vi "Open.vi"(7 "Config data in":variant, 8 "error in (no error)":errorcluster, 9 "Timeout (ms)":u32=3000, 10 "VISA session":refnum<visa-resource-name>="TCPIP::146.201.232.88::7180::SOCKET", 11 "PS Driver.lvlib:PS Driver.lvclass in":refnum<class "PS Driver.lvclass">) -> (0 "error out":errorcluster, 1 "Config data out":variant, 2 "dup VISA Session":refnum<visa-resource-name>, 3 "PS Driver.lvlib:PS Driver.lvclass out":refnum<class "PS Driver.lvclass">)   [LabVIEW 2020, in "PS Driver.lvlib" / "PS Driver.lvclass"]
uses:
  PS Driver.lvclass
  PS Driver.lvclass/PS Driver.ctl
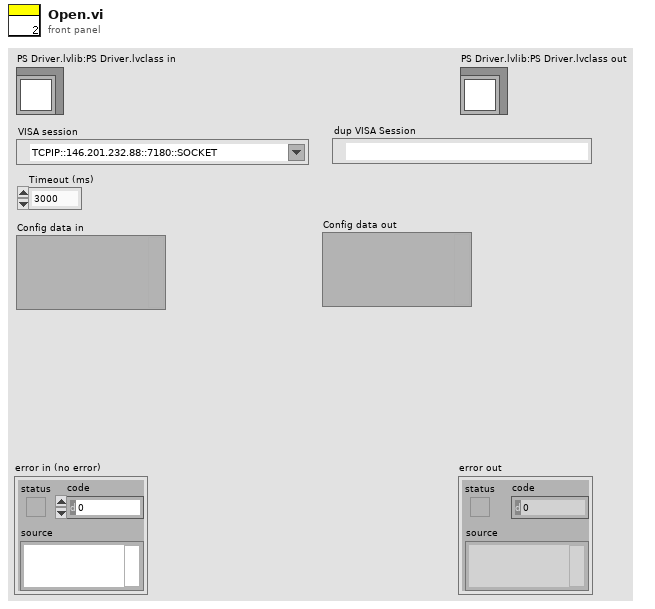
[diagram p1: front panel]
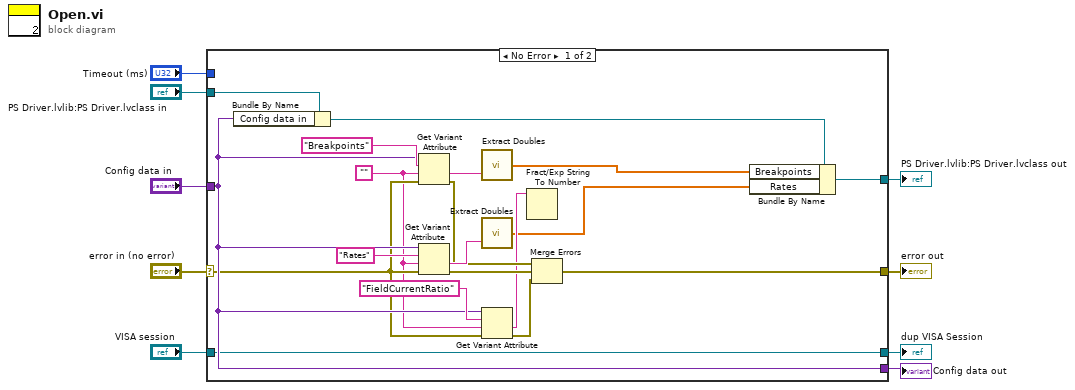
[diagram p0: block diagram]
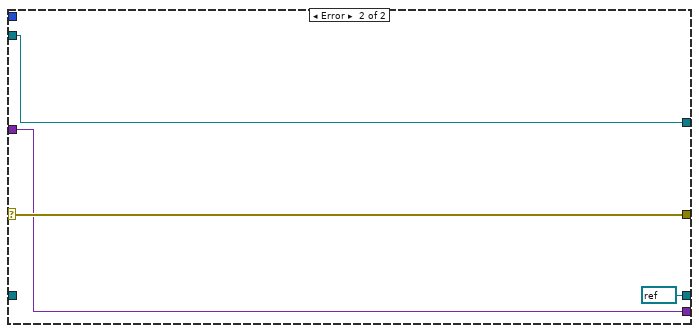
[diagram p2: hidden frame]
diagram:
  n1 = case shown="No Error" "error in (no error)" {
    selector: "error in (no error)" -> [w16 w32]
    tunnel: [w20 w32] -> w8
    tunnel: [w19 w31] -> w6
    tunnel: "PS Driver.lvlib:PS Driver.lvclass in" -> [w28 w31]
    tunnel: "VISA session" -> [w12 _]
    tunnel: "Timeout (ms)" -> [_ _]
    tunnel: "Config data in" -> [w17 w29]
    tunnel: [w12 refnum<visa-resource-name> refnum ("dup VISA Session")] -> w2
    tunnel: [w17 w29] -> w1
    frame No Error {
      w14 = ""
      n2 = Bundle By Name(cluster=w28, "Config data in"=w17) -> (w23:refnum<class "PS Driver.lvclass">)
      n3 = Get Variant Attribute(Variant=w17, name="Breakpoints", default value (empty Variant)=w14, error in=w16) -> (value=w25:string, error out=w22:errorcluster)  [unwired: 2 out]
      n4 = Get Variant Attribute(Variant=w17, name="Rates", default value (empty Variant)=w14, error in=w16) -> (value=w24:string, error out=w21:errorcluster)  [unwired: 2 out]
      n5 = call "Extract Doubles.vi"("String"=w25) -> ("Data"=w11:dbl[])  [unwired: 1 in]
      n6 = call "Extract Doubles.vi"("String"=w24) -> ("Data"=w10:dbl[])  [unwired: 1 in]
      n7 = Get Variant Attribute(Variant=w17, name="FieldCurrentRatio", default value (empty Variant)=w14, error in=w16) -> (value=w13:string, error out=w15:errorcluster)  [unwired: 2 out]
      n8 = Fract/Exp String To Number(string=w13) -> ()  [unwired: 3 in, 2 out]
      n9 = Merge Errors(w22, w21, w15) -> (w20:errorcluster)
      n10 = Bundle By Name(cluster=w23, "Breakpoints"=w11, "Rates"=w10) -> (w19:refnum<class "PS Driver.lvclass">)
    }
    frame Error {
    }
  }
  "error out" <- w8
  "PS Driver.lvlib:PS Driver.lvclass out" <- w6
  "dup VISA Session" <- w2
  "Config data out" <- w1
